vi "CO Monitor Troubleshooting.vi"() -> ()   [LabVIEW 2014]
panel:
  out "CO Monitor Troubleshooting":string="For normal calibration operation, the CO concentration should reach a nominal CO value of around 500ppb and then reach to a zero ppb value. In the event that the front Amber LED does not lit or it does NOT reach to the zero ppb, after the calibration has finished, on the instrument touch screen, press \n\n1.\tShift F5 -> Calibration -> Start -> Yes (calibration will fail again which is Ok)\n2.\tShift F5 -> Calibration -> Start -> Yes (calibration should work with amber LED lit).\n\nThis should have rectified the fault due to the internal calibration software.  \n"
  in  "Exit":bool
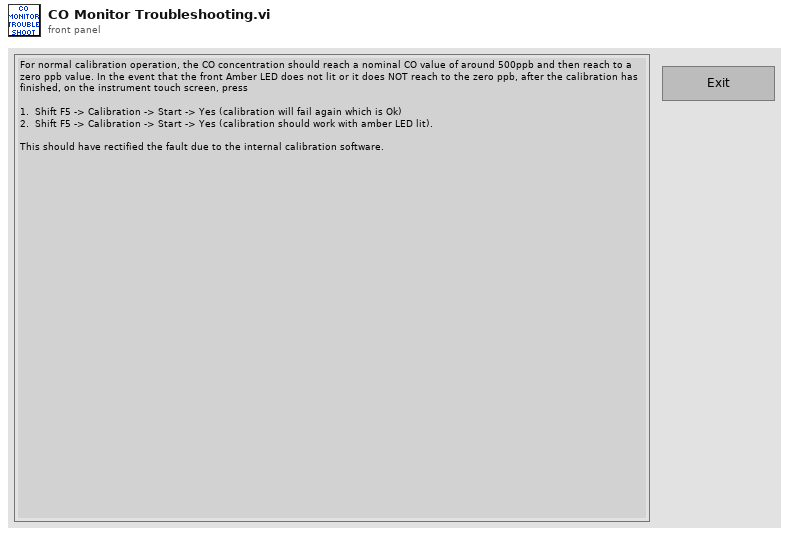
[diagram p1: front panel]
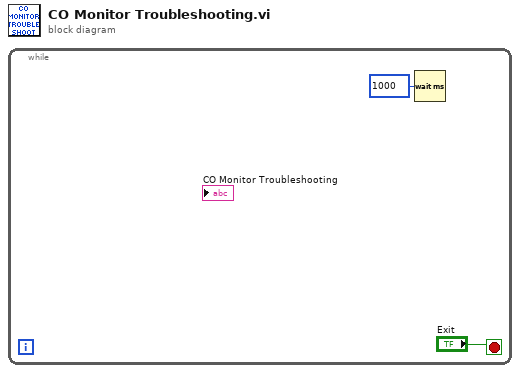
[diagram p0: block diagram]
diagram:
  n1 = while {
    stop <- "Exit" stop-if-true
    n2 = Wait (ms)(milliseconds to wait=u32 1000) -> ()  [unwired: 1 out]
  }
